vi "arm encoder location.vi"() -> (7 "Encoder Distance":dbl)   [LabVIEW 2014]
uses:
  global variables/devrefs.vi
panel:
  # "A Space Saving VI"
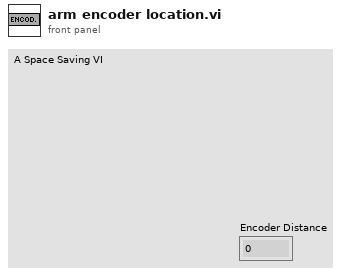
[diagram p1: front panel]
types:
  T1 = typedef "WPI_EncoderDevRef.ctl" = cluster{"DevStatus":errorcluster, "EncoderIndex":T2, "CounterIndex":T3, "DistancePerCount":dbl, "Decoding Type":T4}
  T2 = typedef "FPGA_EncoderIdx.ctl" = enum8{"Enc 0", "Enc 1", "Enc 2", "Enc 3", "Enc 4", "Enc 5", "Enc 6", "Enc 7", "Invalid"}
  T3 = typedef "FPGA_CounterCtrSystemIndex.ctl" = enum8{"Ctr 0", "Ctr 1", "Ctr 2", "Ctr 3", "Ctr 4", "Ctr 5", "Ctr 6", "Ctr 7", "Invalid"}
  T4 = typedef "WPI_EncoderType.ctl" = enum16{"1x", "2x", "4x"}
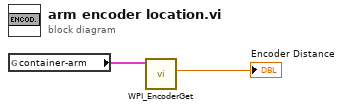
[diagram p0: block diagram]
diagram:
  n1 = global read "devrefs.vi" "container-arm"() -> (w2:T1)
  n2 = call <vilib>:"WPI_EncoderGet.vi"("EncoderDevRef"=w2) -> ("Distance"=→"Encoder Distance":dbl)  [unwired: 5 in, 5 out]
